vi "matrici_v30.vi"() -> ()   [LabVIEW 2009]
uses:
  <vilib>/Analysis/Matrix/Datatypes/RealMatrix.ctl
  <vilib>/Analysis/Matrix/NI_Matrix.lvlib
panel:
  in  "stop":bool
  out "Real Matrix":T1=[[96.31435578380301, 13.563751169243154, 56.621862158126326, 39.12846510797971, 88.30662777084059, 49.74896217151932, 77.89478314685263], [52.68345806259016, 41.262861321520546, 1.0652803786199705, 83.41926112491575, 2.6776393775314933, 13.708915759775087, 87.1873327297392], [57.586643940739265, 21.902129184874262, 71.35450746862162, 29.455429749391193, 72.54083765809585, 15.764649289670416, 86.86818810267367], [46.73949376432962, 3.197882029626342, 73.8823790686913, 15.454457998928795, 56.14370254906653, 56.39344484928772, 0.13516237538486742], [82.06266396988026, 21.416955629163816, 3.172891251699017, 91.86747070568286, 30.470134665553815, 16.08798469552135, 80.21025961459863]]
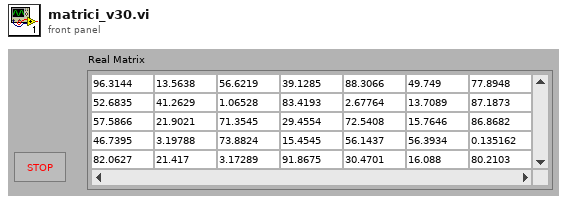
[diagram p1: front panel]
types:
  T1 = typedef "NI_Matrix.lvlib/RealMatrix.ctl" = dbl[][]
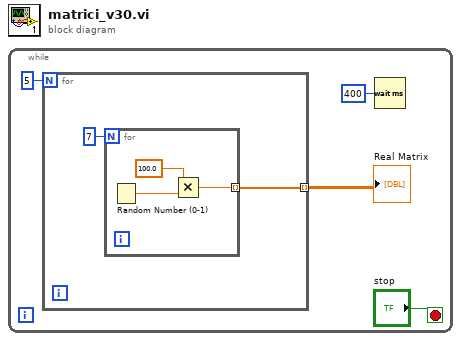
[diagram p0: block diagram]
diagram:
  n1 = while {
    stop <- "stop" stop-if-true
    n2 = for {
      N: 5 -> [_]
      tunnel: [w5] -> w3 mode=indexing
      n3 = for {
        N: 7 -> [_]
        tunnel: [w8] -> w5 mode=indexing
        n4 = Random Number (0-1)() -> (number: 0 to 1=w9:dbl)
        n5 = Multiply(x=100.0, y=w9) -> (x*y=w8:dbl)
      }
    }
    "Real Matrix" <- w3
    n6 = Wait (ms)(milliseconds to wait=u32 400) -> ()  [unwired: 1 out]
  }
